vi "Read Waveforms.vi"(8 "error in (no error)":errorcluster, 10 "data (all)":u16(ring)=2 items=["voltage", "current", "all"], 11 "VI Probe in":refnum<class "PL MKS VI Probe.lvclass">) -> (0 "error out":errorcluster, 2 "waveforms":T1, 3 "VI Probe out":refnum<class "PL MKS VI Probe.lvclass">)   [LabVIEW 2015, in "PL MKS VI Probe.lvclass"]
doc: "Reads waveforms."
uses:
  PL MKS VI Probe.lvclass
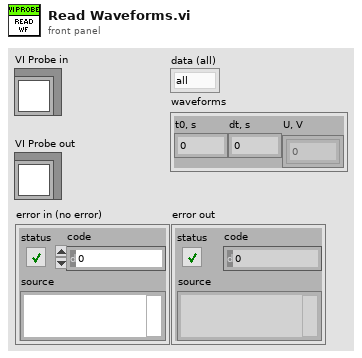
[diagram p1: front panel]
types:
  T1 = cluster{"t0, s":dbl, "dt, s":dbl, "U, V":dbl[][]}
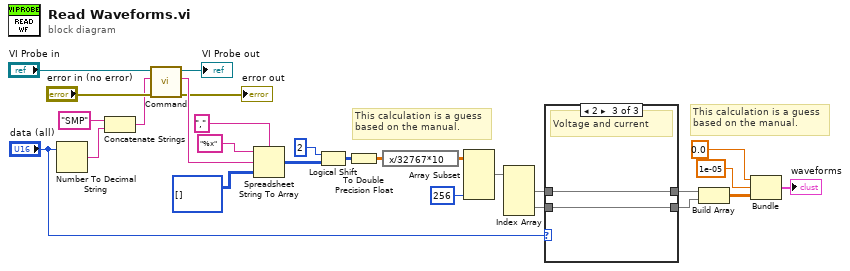
[diagram p0: block diagram]
diagram:
  # "This calculation is a guess\nbased on the manual."
  # "This calculation is a guess\nbased on the manual."
  n1 = Number To Decimal String(number="data (all)") -> (decimal integer string=w24:string)  [unwired: 1 in]
  n2 = Concatenate Strings("SMP" ("format string"), w24) -> (w22:string)
  n3 = call "Command.vi"("error in (no error)"="error in (no error)", "command"=w22, "VI Probe in"="VI Probe in") -> ("error out"=→"error out":errorcluster, "response data"=w18:string, "VI Probe out"=→"VI Probe out":refnum<class "PL MKS VI Probe.lvclass">)  [unwired: 6 in]
  n4 = Spreadsheet String To Array(delimiter (Tab)="," ("format string"), format string="%x", spreadsheet string=w18, array type (2D Dbl)=i16[][] []) -> (array=w11:i16[][])
  n5 = Logical Shift(y=i16 2, x=w11) -> (x << y=w5:i16[][])
  n6 = To Double Precision Float(number=w5) -> (double precision float=w7:dbl[][])
  n7 = expression code="x/32767*10"(w7) -> (w6:dbl[][])
  n8 = Array Subset(array=w6, length (col)=256 ("length")) -> (w14:dbl[][])  [unwired: 3 in]
  n9 = Index Array(array=w14) -> (element #1=w13:dbl[], element #2=w12:dbl[])  [unwired: 4 in]
  n10 = case shown="2" "data (all)" {
    tunnel: w13 -> [w28 w29 w31]
    tunnel: w12 -> [_ _ w30]
    tunnel: [w28 _ w31] -> w4
    tunnel: [_ w29 w30] -> w3
    frame 0, Default {
      # "Voltage"
    }
    frame 1 {
      # "Current"
    }
    frame 2 {
      # "Voltage and current"
    }
  }
  n11 = Build Array(w4, w3) -> (w1:dbl[][])
  n12 = Bundle(0.0, 1e-05, w1) -> (→"waveforms":cluster{dbl, dbl, dbl[][]})  [unwired: 1 in]
